vi "Read and Unflatten.vi"(8 "error in (no error)":errorcluster, 9 "Timeout (ms)":i32, 10 "Data in":T2[](array[typedef]), 11 "CIF_NIChn_FIFO_DAQ in":refnum<class "CIF_NIChn_FIFO_DAQ.lvclass">) -> (0 "error out":errorcluster, 1 "Timed out?":bool, 2 "Data out":T2[](array[typedef]), 3 "CIF_NIChn_FIFO_DAQ out":refnum<class "CIF_NIChn_FIFO_DAQ.lvclass">, 4 "Header out":T1)   [LabVIEW 2021, in "CIF_NIChn_FIFO_DAQ.lvclass"]
uses:
  CIF_NIChn_FIFO_DAQ.lvclass
  D:/dev/Packages/Channel_Manager/src/CIF_NIChn/NIChn/CIF_NIChn.lvclass
  D:/dev/Packages/Channel_Manager/src/CIFChannels/CIFChannels.lvclass
  ChannelCommon/typedef/Datatype Waveform.ctl
  ChannelCommon/typedef/FIFO Header.ctl
  NIChn/CIF_NIChn.lvclass/CIF_NIChn.ctl
  CIFChannels/CIFChannels.lvclass/CIFChannels.ctl
  <vilib>/CIF Foundation/CIF Utilities/Statistics/I64/Stats_I64_CIF_U.lvclass/Stats_I64_CIF_U.ctl
  8d434fcd-ba02-44c6-a1d2-d54d1c5f4ff9.vi
  c632fbd8-b242-46ac-b145-31e81b296fef.vi
  ChannelCommon/Utilities/Add Error.vi
  <vilib>/CIF Foundation/CIF Channels/CIFChannels/Top Level/Read U8 Array.vi/4bc1c15b-36ab-481f-b8dd-c64075ce723a.vi
  <vilib>/CIF Foundation/CIF Channels/CIFChannels/Top Level/Read U8 Array.vi/d83cb72b-7713-41fc-a3d1-682de79cf574.vi
  <vilib>/CIF Foundation/CIF Channels/CIFChannels/SubVIs/Get dll Path.vi
  <vilib>/CIF Foundation/CIF Channels/CIFChannels/SubVIs/Get Requested Size.vi
  <vilib>/CIF Foundation/CIF Channels/CIFChannels/Top Level/Advanced/Read U8 FIFO as Dbl Array.vi/4bc1c15b-36ab-481f-b8dd-c64075ce723a.vi
  <vilib>/CIF Foundation/CIF Channels/CIFChannels/Top Level/Advanced/Read U8 FIFO as Dbl Array.vi/d83cb72b-7713-41fc-a3d1-682de79cf574.vi
  <vilib>/CIF Foundation/CIF Utilities/Statistics/I64/X1 minus X0.vi
  <vilib>/CIF Foundation/CIF Utilities/Time/System Time/Get System Time.vi
  <vilib>/CIF Foundation/CIF Utilities/Errors/Append Error Location.vi
  <vilib>/CIF Foundation/CIF Utilities/Statistics/I64/X1 minus X0.vi/dfabcf33-0dbc-4041-80a5-3dc0c86d2989.vi
  <vilib>/CIF Foundation/CIF Utilities/Time/System Time/LabVIEW Time to TAI Time.vi
  <vilib>/CIF Foundation/CIF Utilities/Statistics/I64/X1 minus X0.vi/dfabcf33-0dbc-4041-80a5-3dc0c86d2989.vi/9eb60a9a-770f-4d2d-8b3f-8465c267ecc9.vi
  NIChn/CIF_NIChn.lvclass
  ChannelCommon/ChannelCommon.lvlib
  <vilib>/CIF Foundation/CIF Utilities/DataTypes/DataTypes_CIF_U.lvlib
  <vilib>/CIF Foundation/CIF Channels/CIFChannels/CIFChannelCore.lvlib
  CIFChannels/CIFChannels.lvclass
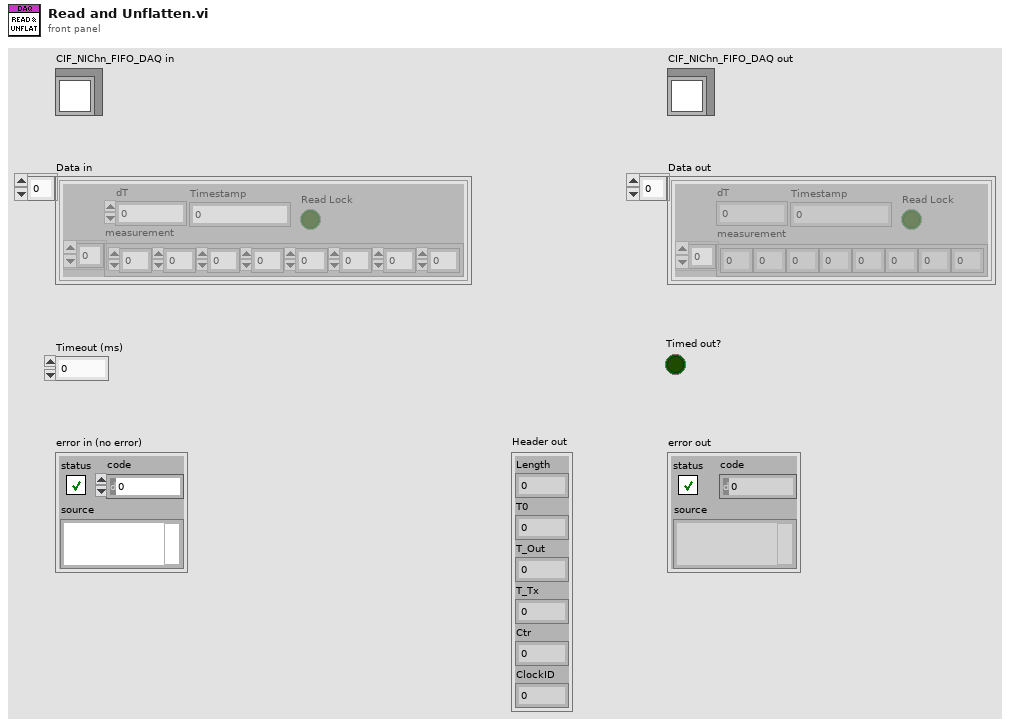
[diagram p1: front panel]
types:
  T1 = typedef "ChannelCommon.lvlib/FIFO Header.ctl" = cluster{"Length":u64, "T0":i64, "T_Out":i64, "T_Tx":i64, "Ctr":u64, "ClockID":u8}
  T2 = typedef "ChannelCommon.lvlib/Datatype Waveform.ctl" = cluster{"measurement":dbl[], "dT":dbl, "Timestamp":i64, "Read Lock":bool}
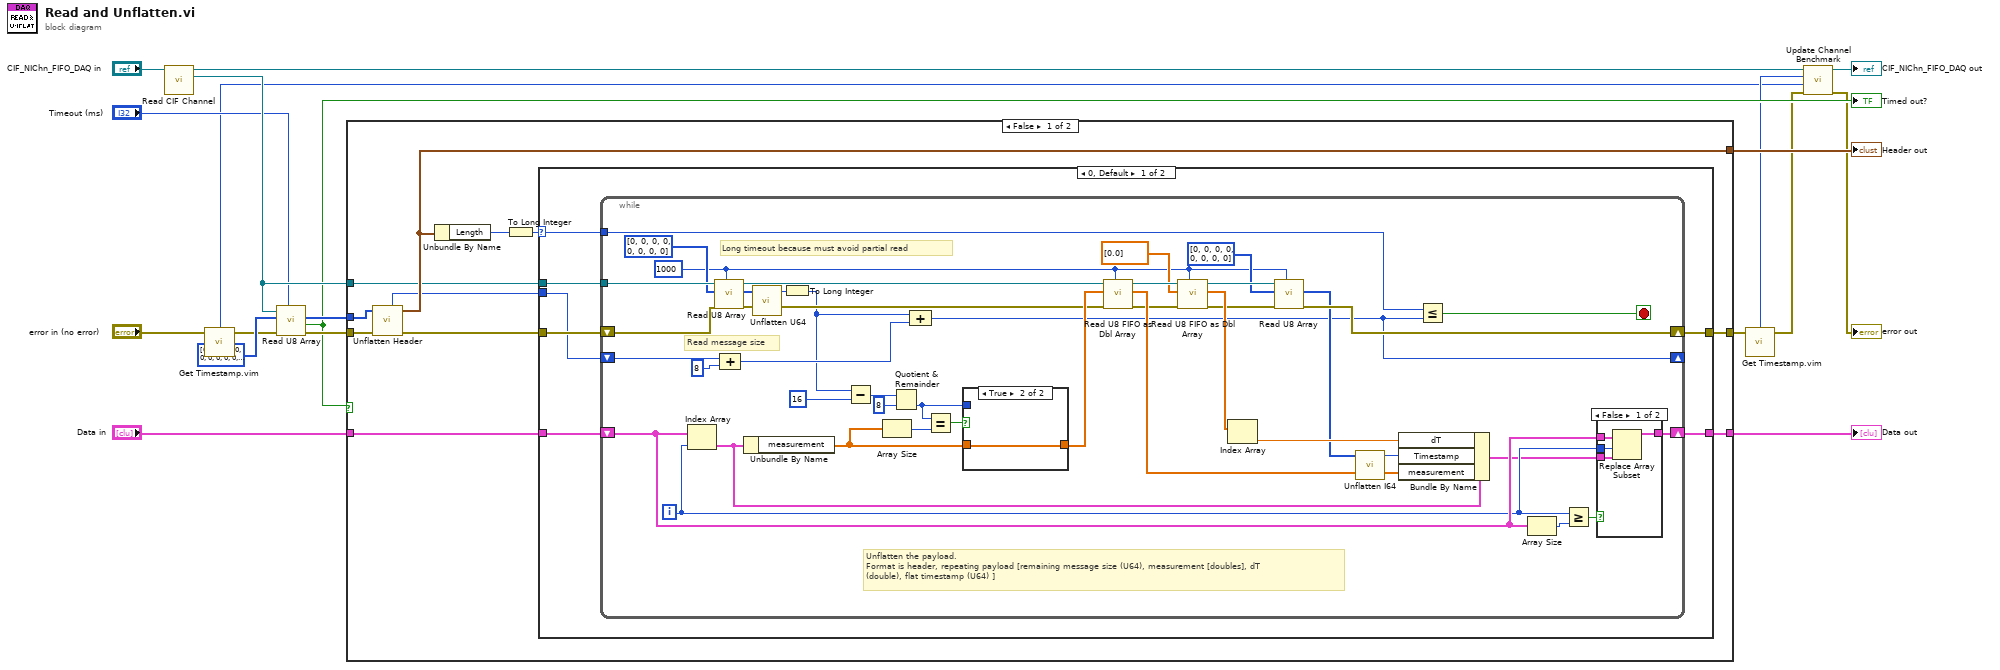
[diagram p0: block diagram]
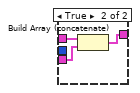
[diagram p2: hidden frame]
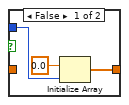
[diagram p3: hidden frame]
diagram:
  n1 = call "Read CIF Channel.vi"("CIFTag in"="CIF_NIChn_FIFO_DAQ in") -> ("CIF Channel"=w13:refnum<k21>, "CIFTag out"=w9:refnum<class "CIF_NIChn_FIFO_DAQ.lvclass">)  [unwired: 8 in, 1 out]
  n2 = call "Get Timestamp.vim"("Anything in"="error in (no error)") -> ("Time (ns)"=w1:i64, "Anything out"=w2:errorcluster)  [unwired: 2 in]
  n3 = call <vilib>:"Read U8 Array.vi"("Timeout (ms)"="Timeout (ms)", "error in"=w2, "U8 Array in"=u8[] [0, 0, 0, 0, 0, 0, 0, 0, 0, 0, 0, 0, 0, 0, 0, 0, 0, 0, 0, 0, 0, 0, 0, 0, 0, 0, 0, 0, 0, 0, 0, 0, 0, 0, 0, 0, 0, 0, 0, 0, 0, 0, 0, 0, 0, 0, 0, 0], "CIF Channel in"=w13) -> ("error out"=w14:errorcluster, "Timed out?"=w12:bool, "U8 Array out"=w15:u8[])  [unwired: 4 in, 1 out]
  "Timed out?" <- w12
  n4 = case shown="False" w12 {
    tunnel: [w30 w93] -> w19
    tunnel: "Data in" -> [w29 w93]
    tunnel: [w26 _] -> w17
    tunnel: w15 -> [w20 _]
    tunnel: w14 -> [w24 w94]
    tunnel: w13 -> [w23 _]
    tunnel: [w22 w94] -> w6
    frame False {
      n5 = call "Unflatten Header.vi"("error in (no error)"=w24, "Flattened Data in"=w20) -> ("error out"=w28:errorcluster, "Header out"=w26:T1, "offset out"=w21:i32)  [unwired: 7 in]
      n6 = Unbundle By Name(w26) -> ("Length"=w27:u64)
      n7 = To Long Integer(number=w27) -> (32bit integer=w25:i32)
      n8 = case shown="0, Default" w25 {
        selector: w25 -> [w33 _]
        tunnel: [w37 w91] -> w30
        tunnel: w29 -> [w36 w91]
        tunnel: [w35 w92] -> w22
        tunnel: w28 -> [w34 w92]
        tunnel: w23 -> [w32 _]
        tunnel: w21 -> [w31 _]
        frame 0, Default {
          n9 = while {
            shift-right: [w77] -> w35
            shift-left: w34 -> [w78]
            shift-right: [w39] -> _
            shift-left: w31 -> [w79]
            tunnel: w33 -> [w76]
            shift-right: [w74] -> w37
            shift-left: w36 -> [w44]
            tunnel: w32 -> [w73]
            i -> [w43]
            stop <- w75 stop-if-true
            w38 = 1000 ("Timeout (ms)")
            # "Long timeout because must avoid partial read"
            # "Read message size"
            # "Unflatten the payload.\nFormat is header, repeating payload [remaining message size (U64), measurement [doubles], dT (double), flat timestamp (U64) ]"
            n10 = Index Array(array=w44, index=w43) -> (element=w72:T2)
            n11 = call <vilib>:"Read U8 Array.vi"("Timeout (ms)"=w38, "error in"=w78, "U8 Array in"=u8[] [0, 0, 0, 0, 0, 0, 0, 0], "CIF Channel in"=w73) -> ("error out"=w57:errorcluster, "U8 Array out"=w61:u8[], "CIF Channel out"=w59:refnum<k21>)  [unwired: 4 in, 1 out]
            n12 = Compound Arithmetic op=ADD(w79, 8 ("value")) -> (w69:i32)
            n13 = Unbundle By Name(w72) -> ("measurement"=w63:dbl[])
            n14 = call <vilib>:"Unflatten U64.vi"("Flat Data"=w61) -> ("U64"=w60:u64)  [unwired: 4 in]
            n15 = To Long Integer(number=w60) -> (32bit integer=w45:i32)
            n16 = Subtract(x=w45, y=16) -> (x-y=w66:i32)
            n17 = Array Size(array=w63) -> (size(s)=w68:i32)
            n18 = Quotient & Remainder(x=w66, y=8) -> (floor(x/y)=w65:i32)  [unwired: 1 out]
            n19 = Compound Arithmetic op=ADD(w45, w69) -> (w39:i32)
            n20 = Equal?(x=w65, y=w68) -> (x = y?=w67:bool)
            n21 = case shown="True" w67 {
              tunnel: w63 -> [_ w90]
              tunnel: [w87 w90] -> w58
              tunnel: w65 -> [w89 _]
              frame False {
                n22 = Initialize Array(0.0, w89) -> (w87:dbl[])
              }
              frame True {
              }
            }
            n23 = call <vilib>:"Read U8 FIFO as Dbl Array.vi"("Timeout (ms)"=w38, "error in"=w57, "DBL Array in"=w58, "CIF Channel in"=w59) -> ("error out"=w54:errorcluster, "DBL Array out"=w56:dbl[], "CIF Channel out"=w55:refnum<k21>)  [unwired: 4 in, 1 out]
            n24 = call <vilib>:"Read U8 FIFO as Dbl Array.vi"("Timeout (ms)"=w38, "error in"=w54, "DBL Array in"=dbl[] [0.0], "CIF Channel in"=w55) -> ("error out"=w46:errorcluster, "DBL Array out"=w52:dbl[], "CIF Channel out"=w50:refnum<k21>)  [unwired: 4 in, 1 out]
            n25 = Index Array(array=w52) -> (element=w51:dbl)  [unwired: 1 in]
            n26 = call <vilib>:"Read U8 Array.vi"("Timeout (ms)"=w38, "error in"=w46, "U8 Array in"=u8[] [0, 0, 0, 0, 0, 0, 0, 0], "CIF Channel in"=w50) -> ("error out"=w77:errorcluster, "U8 Array out"=w48:u8[])  [unwired: 4 in, 2 out]
            n27 = call <vilib>:"Unflatten I64.vi"("Flat Data"=w48) -> ("I64"=w47:i64)  [unwired: 4 in]
            n28 = Bundle By Name(cluster=w72, "dT"=w51, "Timestamp"=w47, "measurement"=w56) -> (w40:T2)
            n29 = Less Or Equal?(x=w76, y=w39) -> (x <= y?=w75:bool)
            n30 = Array Size(array=w44) -> (size(s)=w42:i32)
            n31 = Greater Or Equal?(x=w43, y=w42) -> (x >= y?=w41:bool)
            n32 = case shown="False" w41 {
              tunnel: [w83 w84] -> w74
              tunnel: w40 -> [w82 w85]
              tunnel: w44 -> [w81 w86]
              tunnel: w43 -> [w80 _]
              frame False {
                n33 = Replace Array Subset(array=w81, new element=w82, index=w80) -> (w83:T2[])
              }
              frame True {
                n34 = Build Array (concatenate)(w86, w85) -> (w84:T2[])
              }
            }
          }
        }
        frame 48 {
        }
      }
    }
    frame True {
    }
  }
  "Data out" <- w19
  "Header out" <- w17
  n35 = call "Get Timestamp.vim"("Anything in"=w6) -> ("Time (ns)"=w4:i64, "Anything out"=w5:errorcluster)  [unwired: 2 in]
  n36 = call "Update Channel Benchmark.vi"("error in (no error)"=w5, "X0"=w1, "X1"=w4, "CIFChannels in"=w9) -> ("error out"=→"error out":errorcluster, "CIFChannels out"=→"CIF_NIChn_FIFO_DAQ out":refnum<class "CIF_NIChn_FIFO_DAQ.lvclass">)  [unwired: 6 in]
